vi "data2image_3d.vi"(10 "image_3d":sgl[][][](array[numeric])) -> (2 "image_1d":sgl[](array[numeric]))   [LabVIEW 2014]
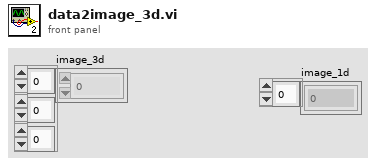
[diagram p1: front panel]
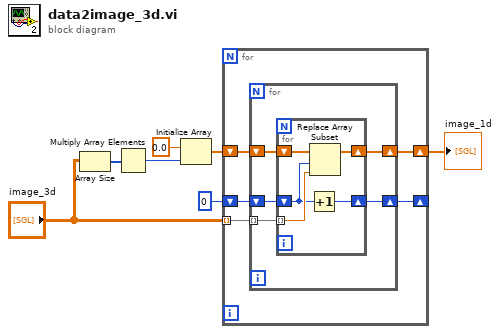
[diagram p0: block diagram]
diagram:
  n1 = Array Size(array="image_3d") -> (size(s)=w3:i32[])
  n2 = Multiply Array Elements(1:w3) -> (0:w4:i32)
  n3 = Initialize Array(sgl 0.0 ("element"), w4) -> (w6:sgl[])
  n4 = for {
    tunnel: "image_3d" -> [w12] mode=indexing
    shift-right: [w11] -> _
    shift-left: 0 -> [w10]
    shift-right: [w8] -> w1
    shift-left: w6 -> [w9]
    n5 = for {
      tunnel: w12 -> [w17] mode=indexing
      shift-right: [w16] -> w11
      shift-left: w10 -> [w15]
      shift-right: [w13] -> w8
      shift-left: w9 -> [w14]
      n6 = for {
        tunnel: w17 -> [w20] mode=indexing
        shift-right: [w22] -> w16
        shift-left: w15 -> [w19]
        shift-right: [w18] -> w13
        shift-left: w14 -> [w21]
        n7 = Increment(x=w19) -> (x+1=w22:i32)
        n8 = Replace Array Subset(array=w21, new element=w20, index=w19) -> (w18:sgl[])
      }
    }
  }
  "image_1d" <- w1
